vi "Create Log File_camera.vi"(8 "error in (no error)":errorcluster, 11 "Acceleration Exceeded Log Folder":path=path "c:/logfiles") -> (0 "error out":errorcluster, 3 "AVI Refnum":T1)   [LabVIEW 2017]
uses:
  <vilib>/vision/Avi.llb/IMAQ AVI2 Refnum.ctl
panel:
  out "appended path":path
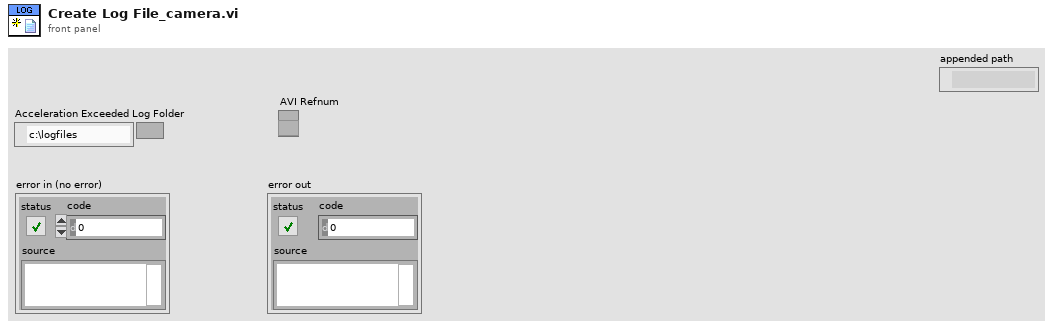
[diagram p1: front panel]
types:
  T1 = typedef "IMAQ AVI2 Refnum.ctl" = refnum<k20>
  T2 = enum16{"open", "open or create", "create or replace", "create", "open (read-only)"}
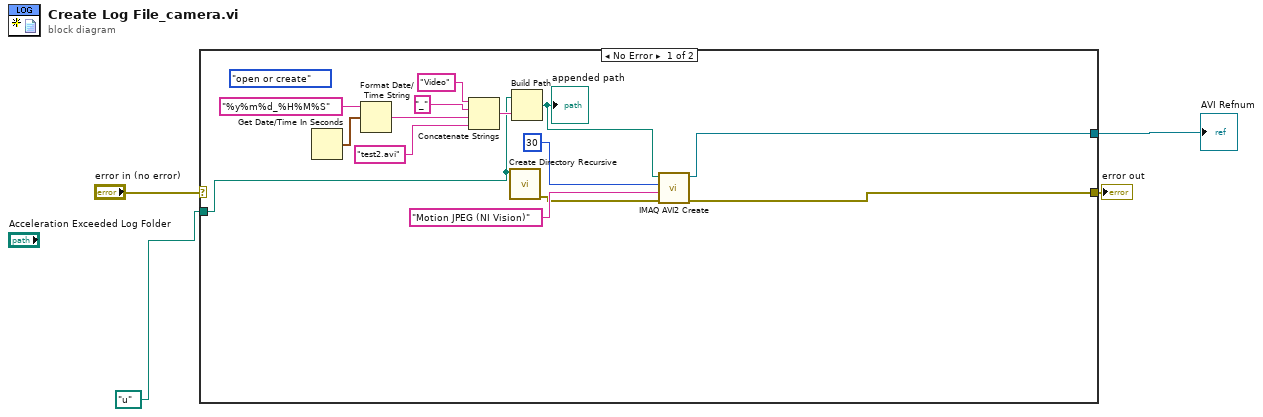
[diagram p0: block diagram]
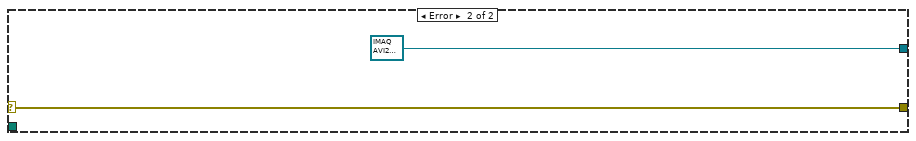
[diagram p2: hidden frame]
diagram:
  n1 = case shown="No Error" "error in (no error)" {
    selector: "error in (no error)" -> [_ w20]
    tunnel: [w8 T1 refnum ("AVI Refnum")] -> w2
    tunnel: path "u:/" ("file path (use dialog)") -> [w10 _]
    tunnel: [w7 w20] -> w3
    frame No Error {
      (unwired) T2."open or create" ("operation (0:open)")
      n2 = Get Date/Time In Seconds() -> (seconds since 1Jan1904=w15:timestamp)
      n3 = Format Date/Time String(time format string (%c)="%y%m%d_%H%M%S", seconds (now)=w15) -> (date/time string=w17:string)  [unwired: 1 out]
      n4 = Concatenate Strings("Video" ("string"), "_" ("string"), w17, "test2.avi" ("name or relative path")) -> (w13:string)
      n5 = call <vilib>:"Create Directory Recursive.vi"("directory"=w10) -> ("error out"=w5:errorcluster)  [unwired: 4 in, 2 out]
      n6 = Build Path(base path=w10, name or relative path=w13) -> (appended path=w6:path)
      "appended path" <- w6
      n7 = call "IMAQ AVI2 Create"("error in (no error)"=w5, "Codec"="Motion JPEG (NI Vision)", "Frames Per Second"=u32 30, "AVI Path"=w6) -> ("error out"=w7:errorcluster, "AVI Refnum"=w8:T1)  [unwired: 6 in]
    }
    frame Error {
    }
  }
  "error out" <- w3
  "AVI Refnum" <- w2
